vi "iLogDemostrator.vi"() -> ()   [LabVIEW 2019]
uses:
  ByteQXAPIBase/TypeDef/Test.ctl
  ByteQXAPIBase/TypeDef/Asset.ctl
  ByteQXAPIBase/TypeDef/Step.ctl
  ByteQXAPIBase/ByteQXAPIBase.lvclass
  ByteQXAPIBase/iLOGAcquisition/Acquisitions.ctl
  <vilib>/numeric/Random Number (Range) U64.vi
  <vilib>/numeric/sub_Random U32.vi
  <vilib>/Bytelabs/ByteSimpleQ/ByteSimpleQ/ByteSimpleQ.lvlib
panel:
  out "Single Asset":string
  in  "Begin Acq":bool
  in  "Channels":cluster{"Channel Name":string, "Delete":bool}[](array[cluster])
  in  "LogSingle":bool
  in  "Asset Code":string="BNC0001"
  in  "Start":bool
  out "Values":cluster{"Channel Name":string, "Value":dbl}[](array[cluster])
  out "Waveform Chart":T1(graph)
  in  "Stop":bool
  out "Title":string
  in  "Channels":cluster{"Channel Name":string, "Delete":bool}[](array[cluster])
  in  "Select Asset":i32(ring) items=["BNC0001"]
  out "InfoStep":string caption="Step Information"
  in  "Select Step":i32(ring) items=["Warm-up"=183, "Full loaded test cycle"=184]
  out "InfoTest":string caption="Test Information"
  in  "Inizia Test":bool
  in  "Select Test":i32(ring) items=["T0008 - Richiesta prova test di durata"=69, "T0003 - Endurance test 19/02/2025"=64, "T0021 - Prova da form"=82, "T0018 - Prova da form"=79, "T0001 - Endurance test 19/02/2025"=62, "T0019 - Prova da form"=80, "T0022 - Test Fan Plan"=83, "T0002 - Endurance test 19/02/2025"=63]
  in  "GetTests":bool
  in  "Starting Date":timestamp format="%<%x>T"
  in  "Workstation":u16(ring) items=["Sala gialla", "POST 1"]
  in  "Exit":bool
  in  "Home":bool
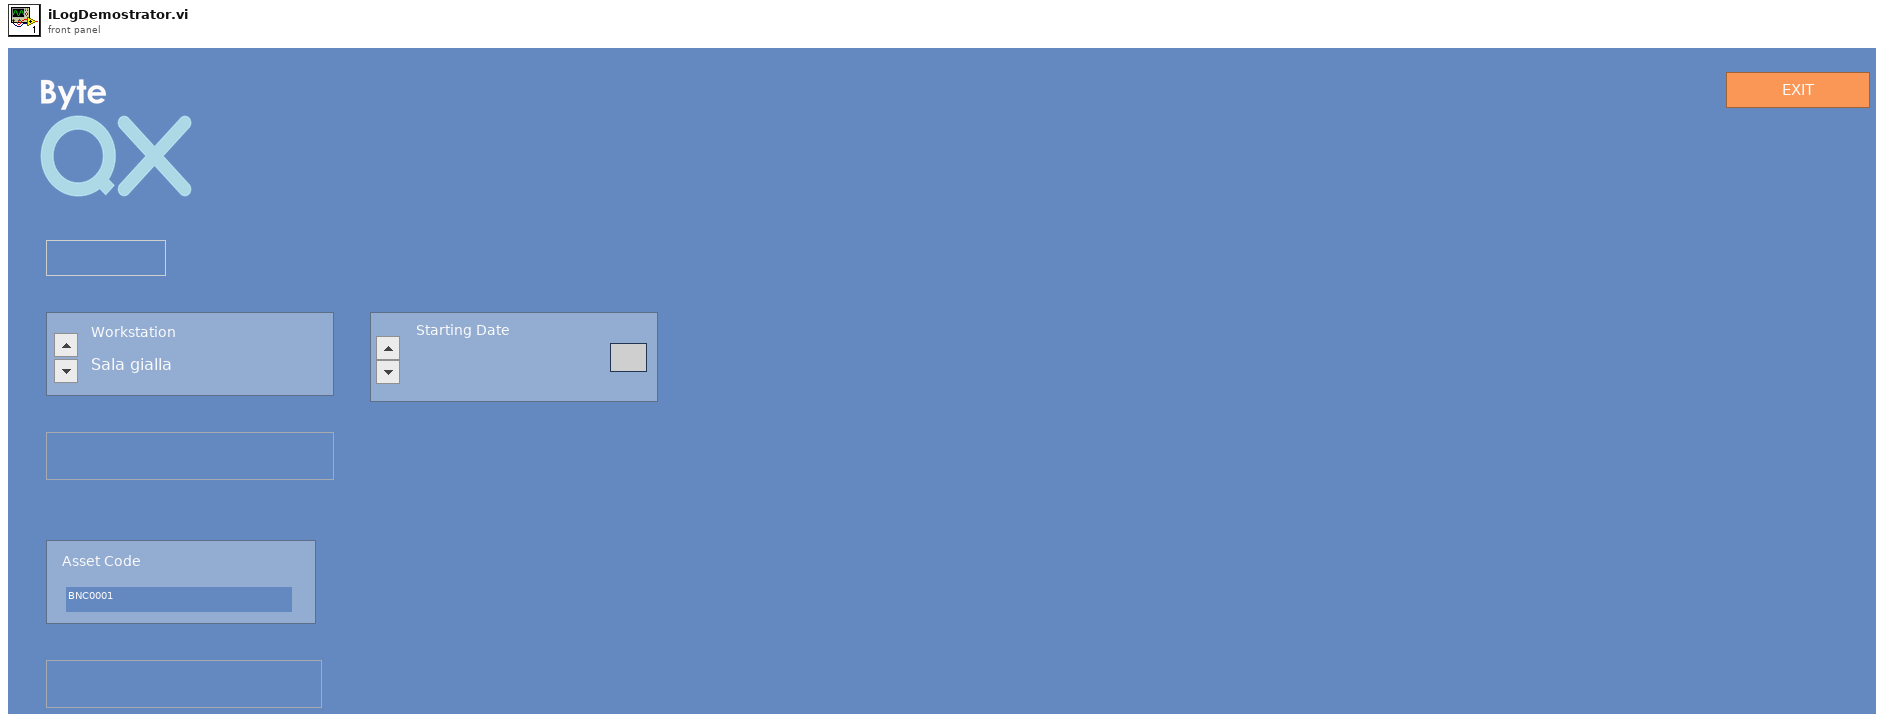
[diagram p1: front panel]
types:
  T1 = cluster{"Graph[0]":u64, "Graph[1]":u64, "Graph[2]":u64, "Graph[3]":u64, "Graph[4]":u64, "Graph[5]":u64, "Graph[6]":u64, "Graph[7]":u64, "Graph[8]":u64, "Graph[9]":u64, "Graph[10]":u64, "Graph[11]":u64, "Graph[12]":u64, "Graph[13]":u64, "Graph[14]":u64, "Graph[15]":u64, "Graph[16]":u64, "Graph[17]":u64, "Graph[18]":u64, "Graph[19]":u64, "Graph[20]":u64, "Graph[21]":u64, "Graph[22]":u64, "Graph[23]":u64, "Graph[24]":u64, "Graph[25]":u64, "Graph[26]":u64, "Graph[27]":u64, "Graph[28]":u64, "Graph[29]":u64, "Graph[30]":u64, "Graph[31]":u64, "Graph[32]":u64, "Graph[33]":u64, "Graph[34]":u64, "Graph[35]":u64, "Graph[36]":u64, "Graph[37]":u64, "Graph[38]":u64, "Graph[39]":u64, "Graph[40]":u64, "Graph[41]":u64, "Graph[42]":u64, "Graph[43]":u64, "Graph[44]":u64, "Graph[45]":u64, "Graph[46]":u64, "Graph[47]":u64, "Graph[48]":u64, "Graph[49]":u64}
  T2 = cluster{"Begin Acq":refnum<vi>, "Channels":refnum<vi>, "Single Asset":refnum<vi>}
  T3 = cluster{"Title":refnum<vi>, "Stop":refnum<vi>, "Values":refnum<vi>, "Start":refnum<vi>, "Waveform Chart":refnum<vi>}
  T4 = typedef "ByteQXWebAPI.lvlib/ByteQXAPIBase.lvclass/Step.ctl" = cluster{"id":i32, "descrizione":string, "prova":cluster{"slug":string}, "assets":T5[], "criterio_accettazione":string, "valore_criterio_accettazione_max":dbl, "valore_criterio_accettazione_min":dbl, "udm_criterio_accettazione":string, "duration_prova":string, "udm_duration_prova":string, "valore_prova":dbl, "ordine":i32, "user":i32, "link_automation":string, "instruction_automation":string, "data_completamento_checklist":timestamp, "outcome":bool, "step_type":string, "channels":string[]}
  T5 = typedef "ByteQXWebAPI.lvlib/ByteQXAPIBase.lvclass/Asset.ctl" = cluster{"descrizione":string, "slug":string, "id":i32}
  T6 = cluster{"Select Test":refnum<vi>, "InfoTest":refnum<vi>, "Inizia Test":refnum<vi>, "Select Step":refnum<vi>, "InfoStep":refnum<vi>, "Select Asset":refnum<vi>, "Channels":refnum<vi>}
  T7 = typedef "ByteQXWebAPI.lvlib/ByteQXAPIBase.lvclass/Test.ctl" = cluster{"titolo":string, "descrizione":string, "statoprova":string, "assets":T5[], "id":i32, "data_apertura_prova":timestamp, "slug":string}
  T8 = cluster{"Workstation":refnum<vi>, "Starting Date":refnum<vi>, "GetTests":refnum<vi>, "Asset Code":refnum<vi>, "LogSingle":refnum<vi>}
  T9 = cluster{"ByteQXAPIBase in":refnum<class "ByteQXAPIBase.lvclass">, "Array dei Test":T7[], "InfoTest":string, "InfoStep":string, "Steps Array":T4[], "queue out":refnum<queue>, "Title":string}
  T10 = cluster{"Single":cluster{"Begin Acq":refnum<vi>, "Channels":refnum<vi>, "Single Asset":refnum<vi>}, "Home":cluster{"Workstation":refnum<vi>, "Starting Date":refnum<vi>, "GetTests":refnum<vi>, "Asset Code":refnum<vi>, "LogSingle":refnum<vi>}, "Test":cluster{"Select Test":refnum<vi>, "InfoTest":refnum<vi>, "Inizia Test":refnum<vi>, "Select Step":refnum<vi>, "InfoStep":refnum<vi>, "Select Asset":refnum<vi>, "Channels":refnum<vi>}, "Running":cluster{"Title":refnum<vi>, "Stop":refnum<vi>, "Values":refnum<vi>, "Start":refnum<vi>, "Waveform Chart":refnum<vi>}}
  T11 = cluster{"Values":cluster{"Channel Name":string, "Value":dbl}[], "ByteQXAPIBase in":refnum<class "ByteQXAPIBase.lvclass">, "slug":string, "Step Id":i32, "AssetCode":string, "Graph":u64[], "Waveform Chart":refnum<vi>}
  T12 = cluster{"Graph[0]":u64, "Graph[1]":u64, "Graph[2]":u64, "Graph[3]":u64, "Graph[4]":u64, "Graph[5]":u64, "Graph[6]":u64, "Graph[7]":u64, "Graph[8]":u64, "Graph[9]":u64, "Graph[10]":u64, "Graph[11]":u64, "Graph[12]":u64, "Graph[13]":u64, "Graph[14]":u64, "Graph[15]":u64, "Graph[16]":u64, "Graph[17]":u64, "Graph[18]":u64, "Graph[19]":u64, "Graph[20]":u64, "Graph[21]":u64, "Graph[22]":u64, "Graph[23]":u64, "Graph[24]":u64, "Graph[25]":u64, "Graph[26]":u64, "Graph[27]":u64, "Graph[28]":u64, "Graph[29]":u64, "Graph[30]":u64, "Graph[31]":u64, "Graph[32]":u64, "Graph[33]":u64, "Graph[34]":u64, "Graph[35]":u64, "Graph[36]":u64, "Graph[37]":u64, "Graph[38]":u64, "Graph[39]":u64, "Graph[40]":u64, "Graph[41]":u64, "Graph[42]":u64, "Graph[43]":u64, "Graph[44]":u64, "Graph[45]":u64, "Graph[46]":u64, "Graph[47]":u64, "Graph[48]":u64, "Graph[49]":u64}[]
  T13 = cluster{"ByteQXAPIBase in":refnum<class "ByteQXAPIBase.lvclass">, "slug":string, "Channels":string[], "Step Id":i32, "AssetCode":string}
  T14 = cluster{"Workstation":u16, "Starting Date":timestamp, "Select Test":i32, "Select Step":i32, "Select Asset":i32, "Channels":cluster{"Channel Name":string, "Delete":bool}[], "Asset Code":string, "Channels":cluster{"Channel Name":string, "Delete":bool}[]}
  T15 = typedef "ByteQXWebAPI.lvlib/ByteQXAPIBase.lvclass/Acquisitions.ctl" = cluster{"timestamp":timestamp, "channels":cluster{"name":string, "value":dbl}[]}
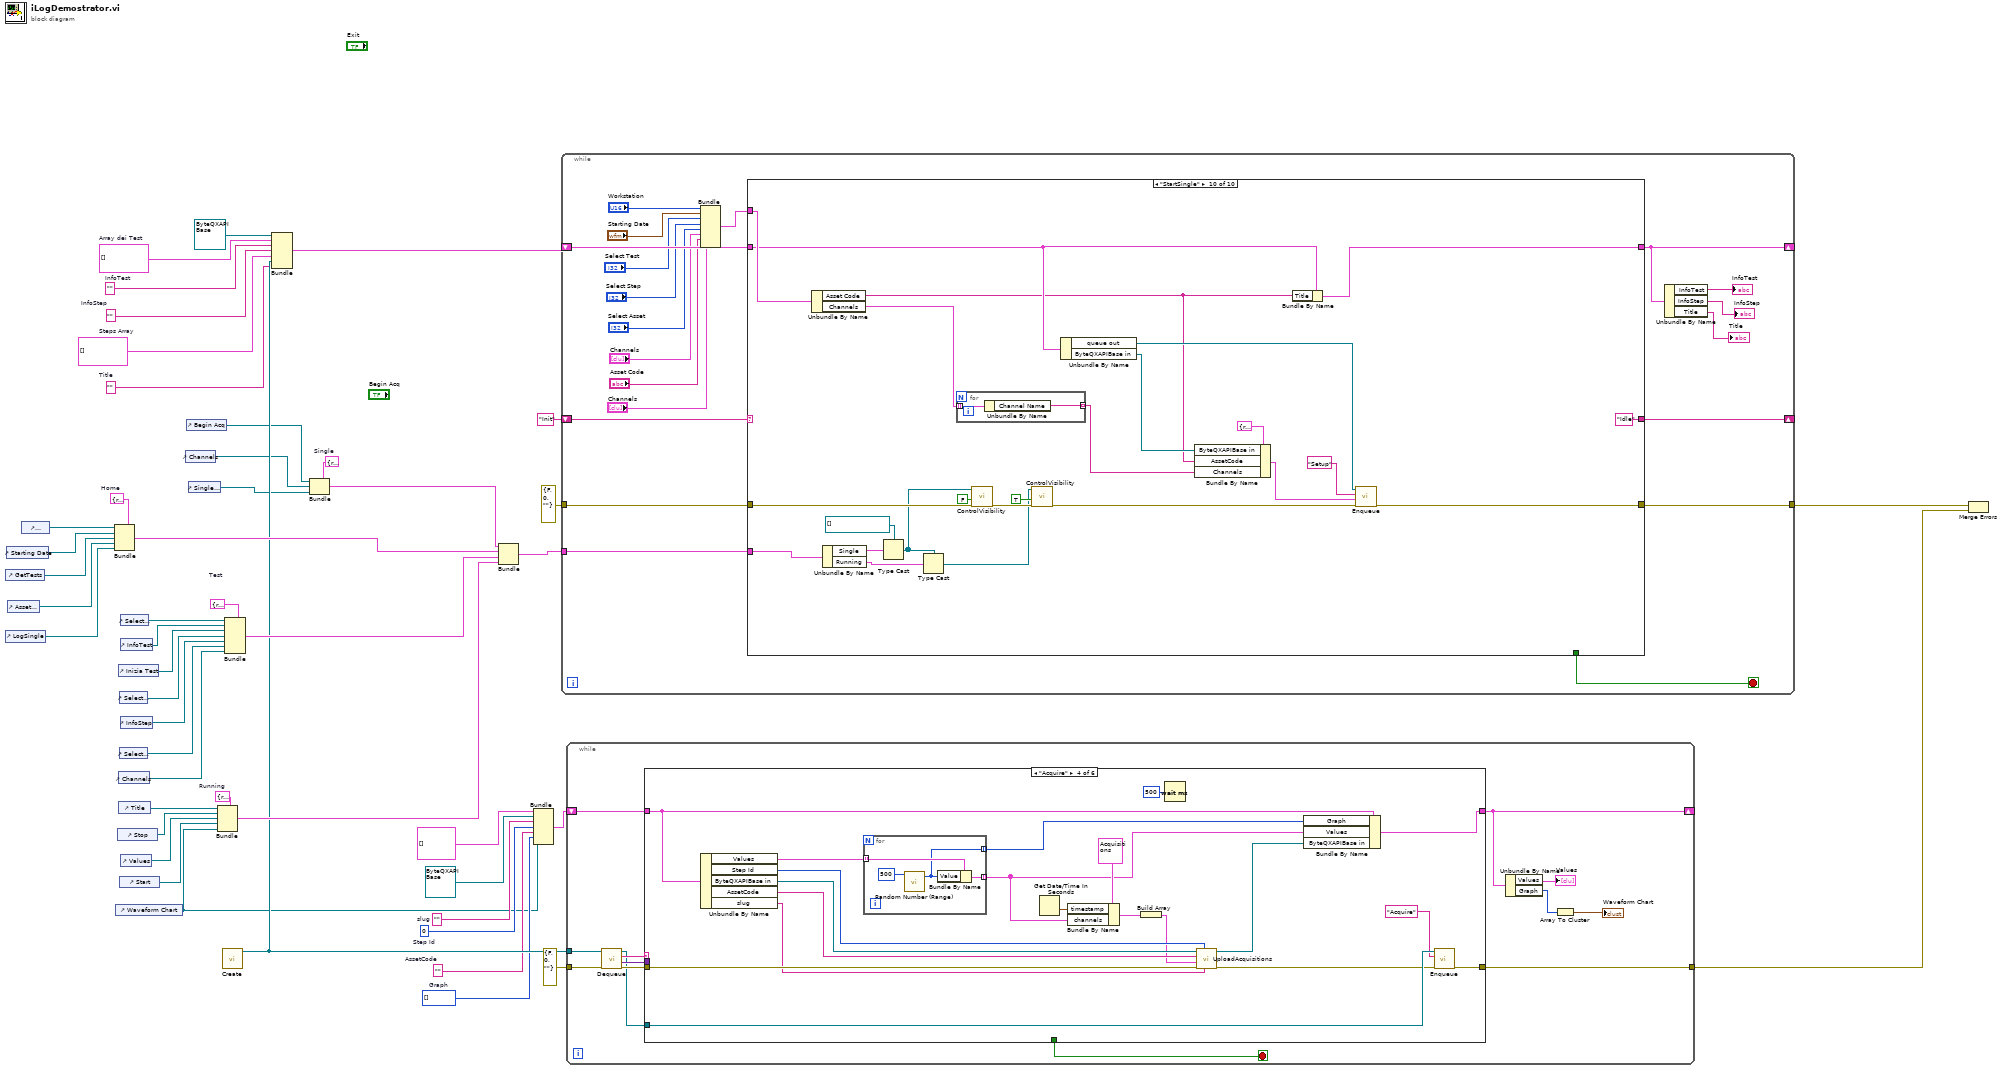
[diagram p0: block diagram]
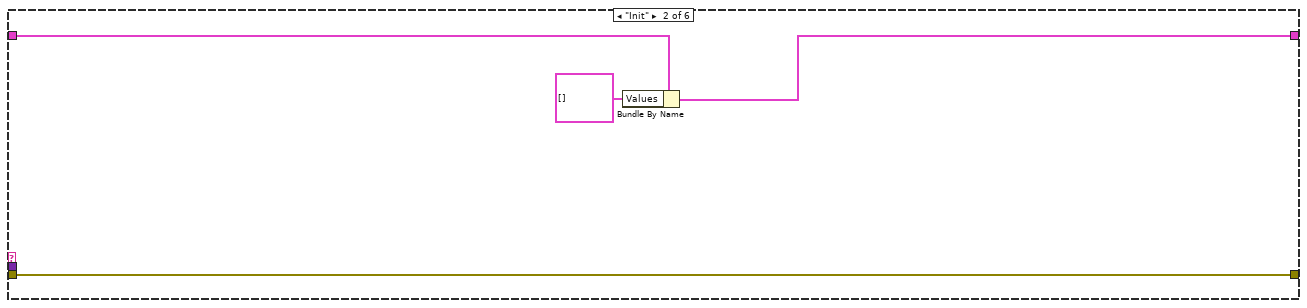
[diagram p3: hidden frame]
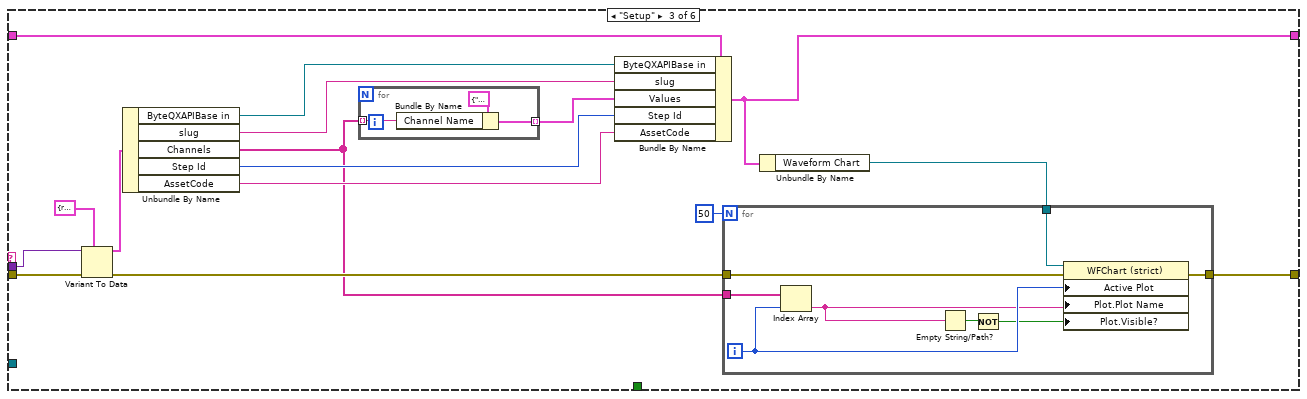
[diagram p4: hidden frame]
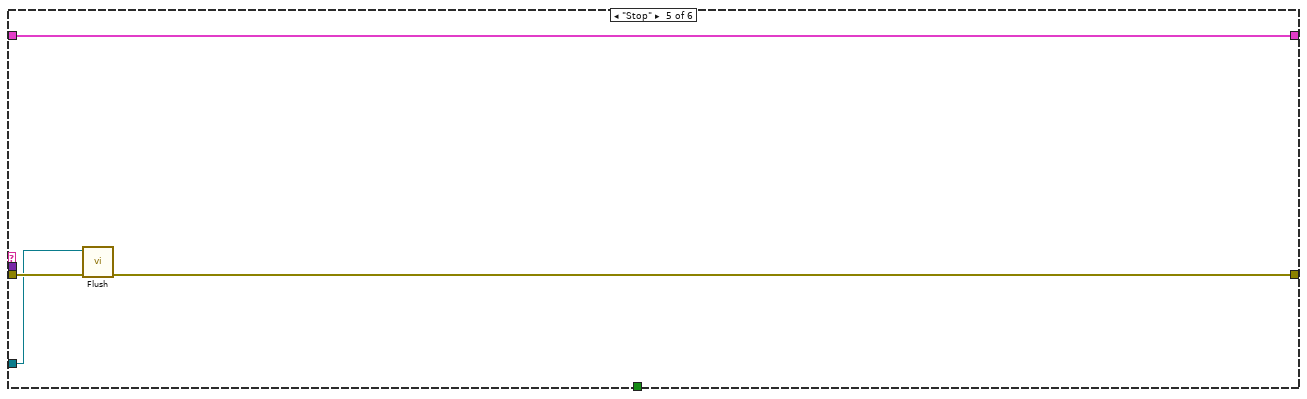
[diagram p5: hidden frame]
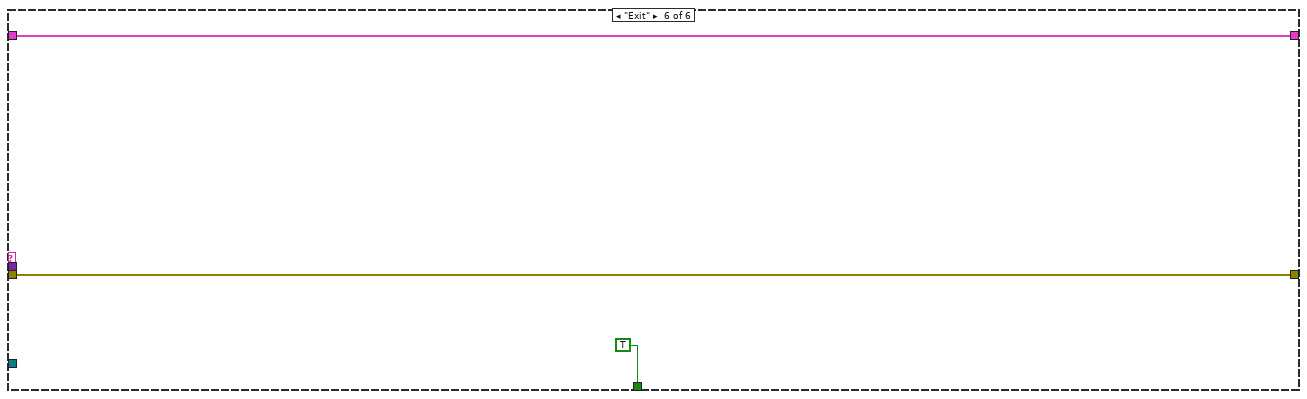
[diagram p6: hidden frame]
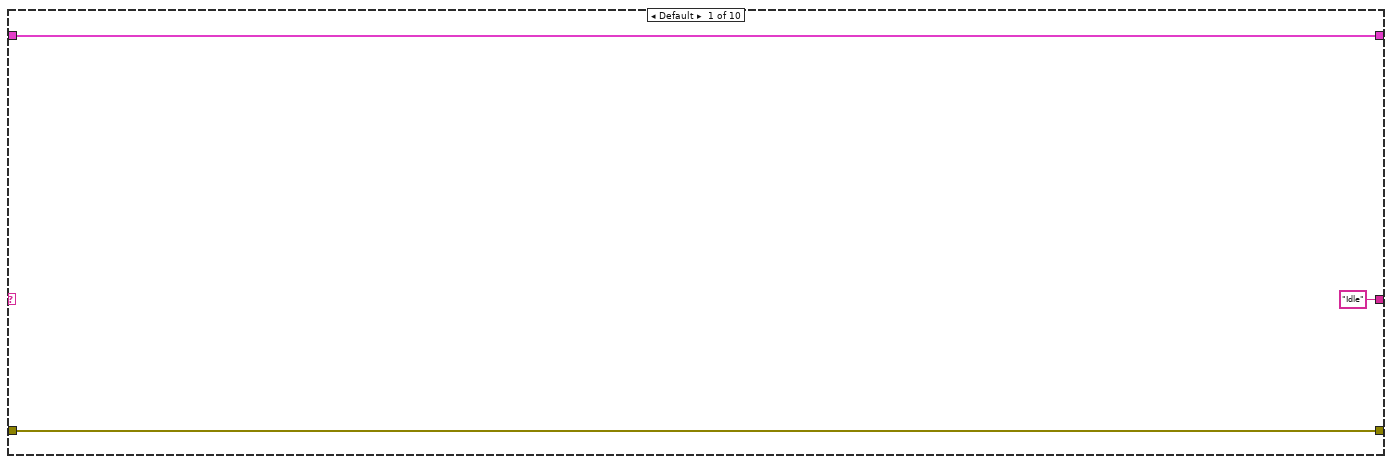
[diagram p7: hidden frame]
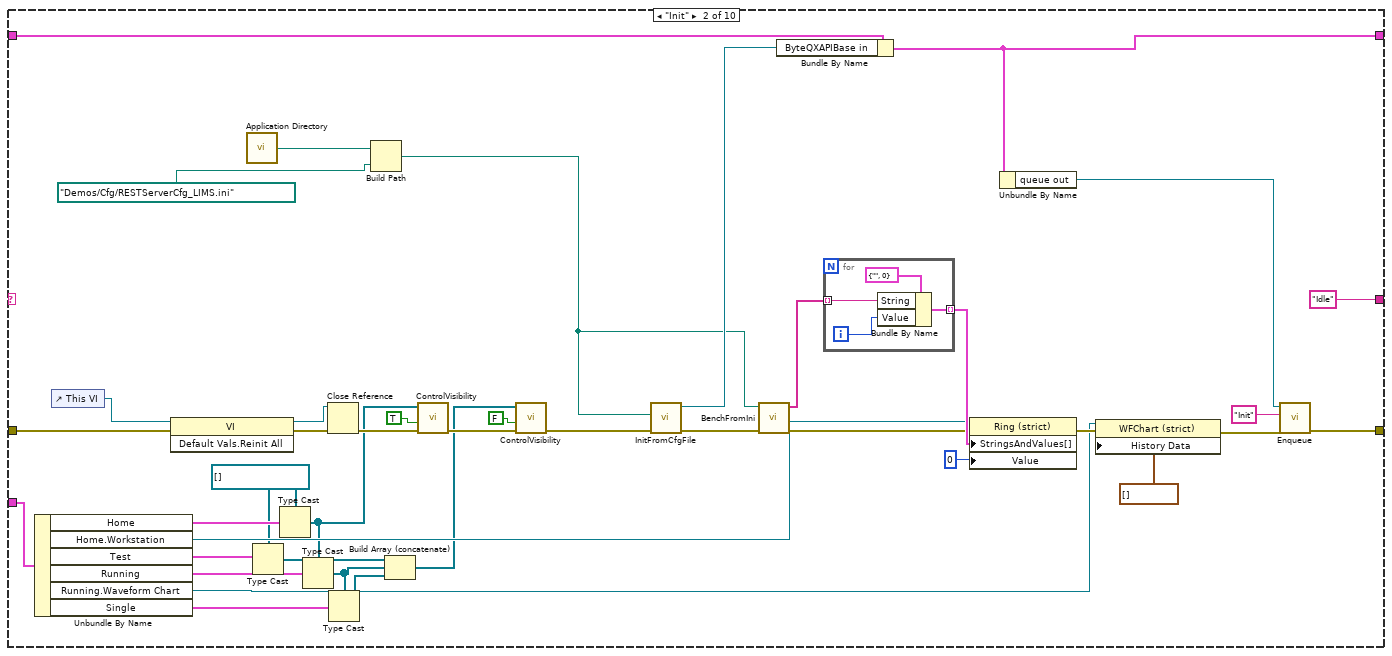
[diagram p8: hidden frame]
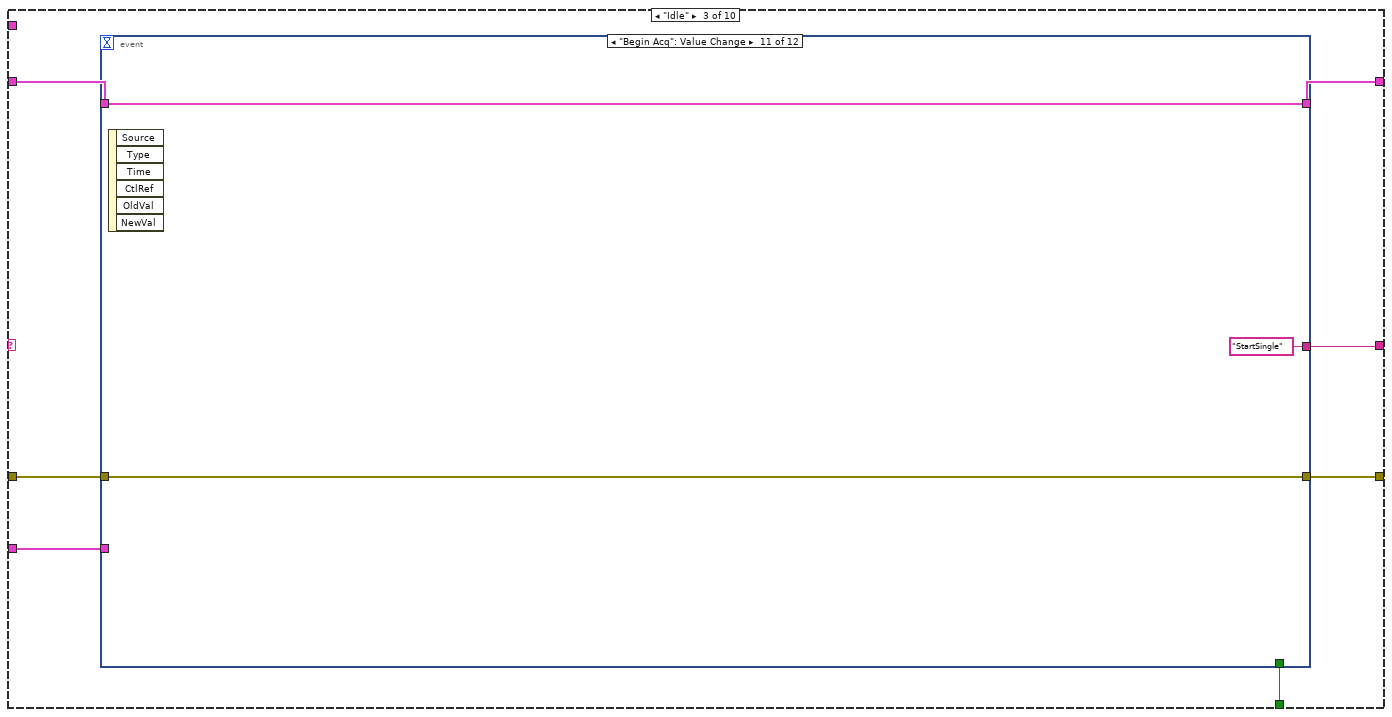
[diagram p9: hidden frame]
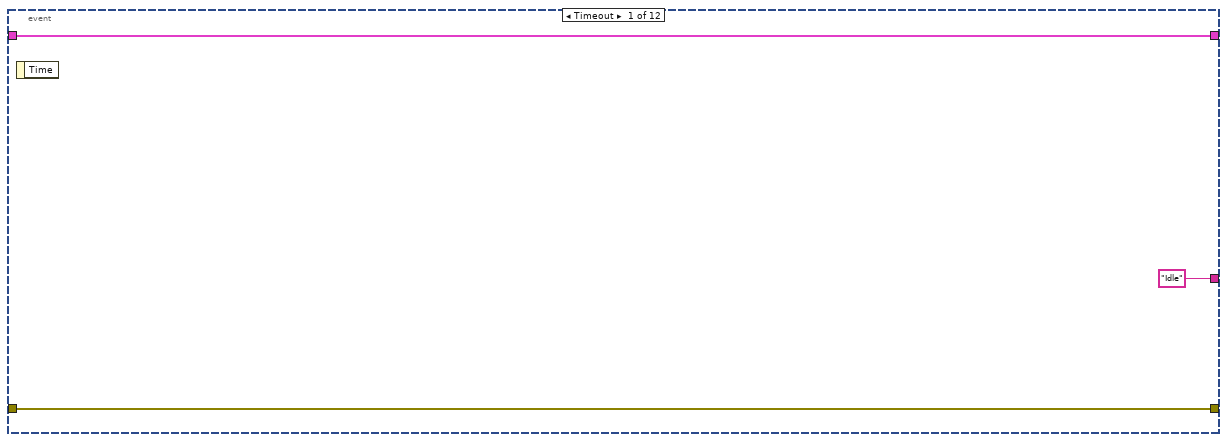
[diagram p10: hidden frame]
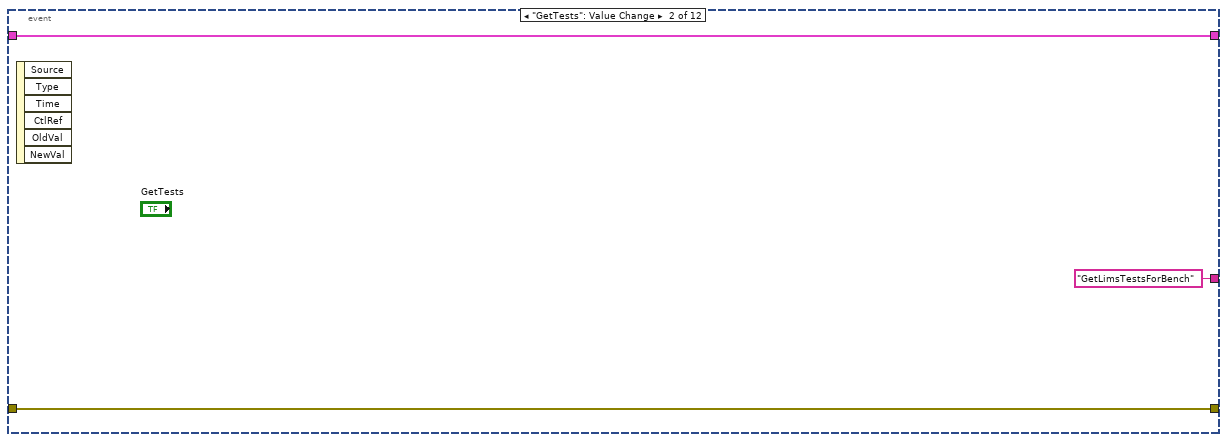
[diagram p11: hidden frame]
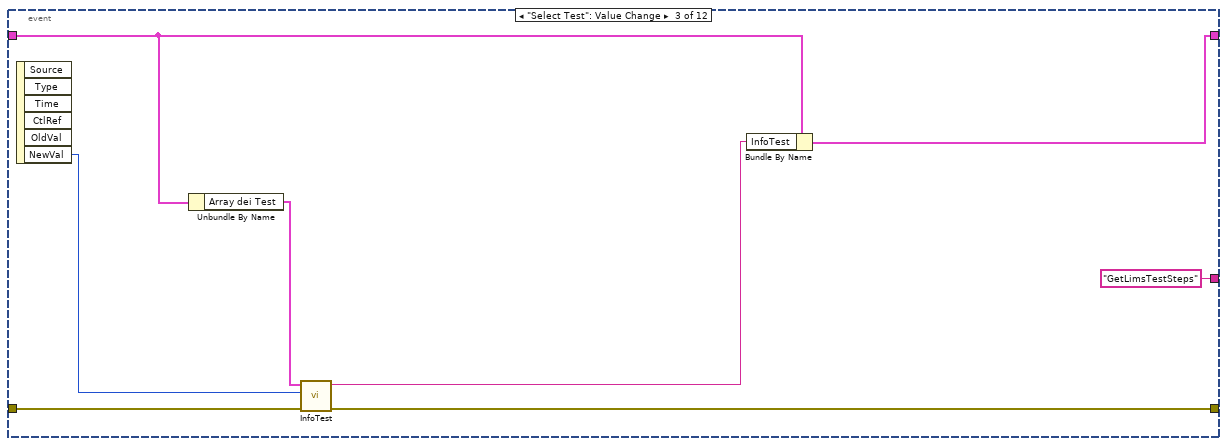
[diagram p12: hidden frame]
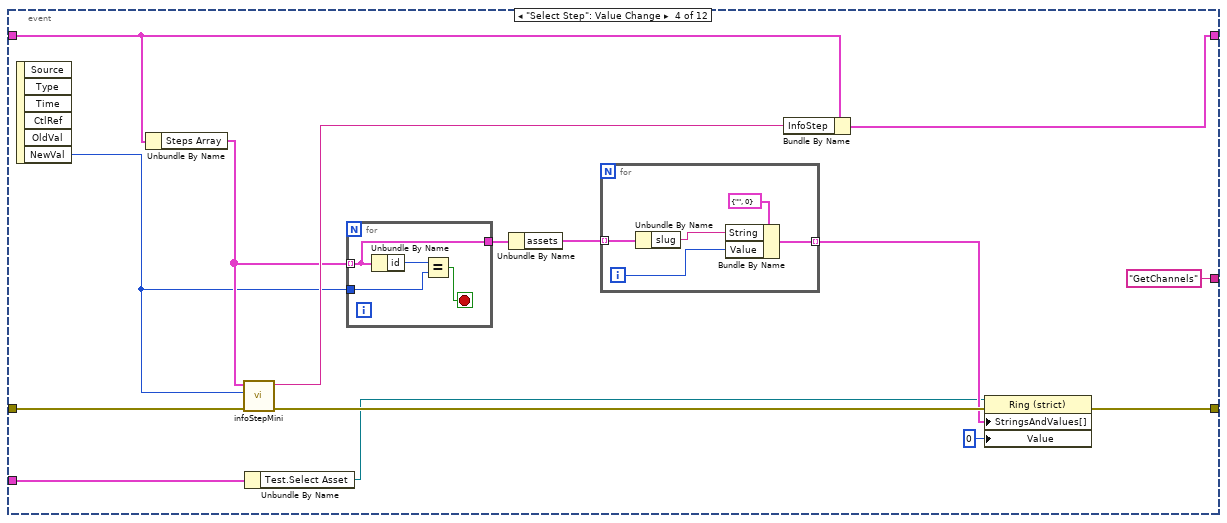
[diagram p13: hidden frame]
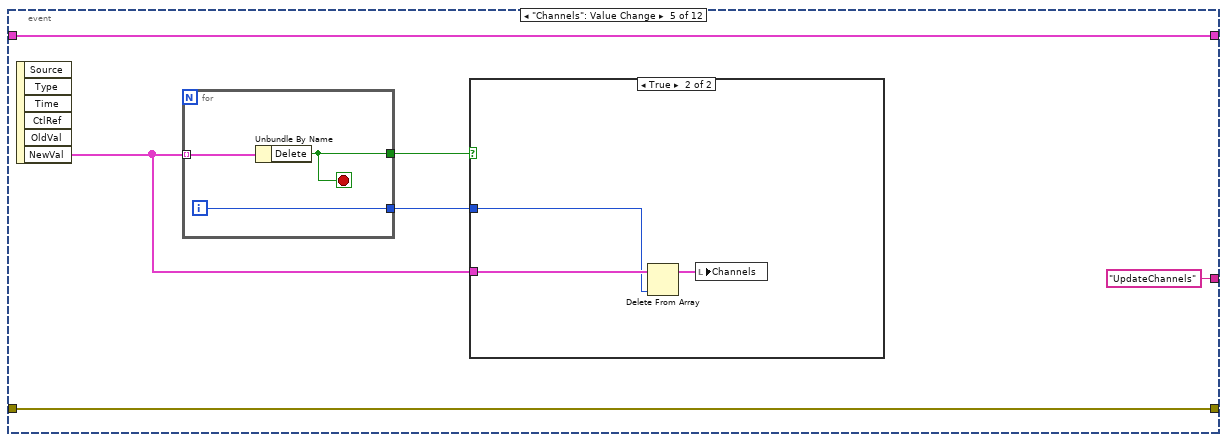
[diagram p14: hidden frame]
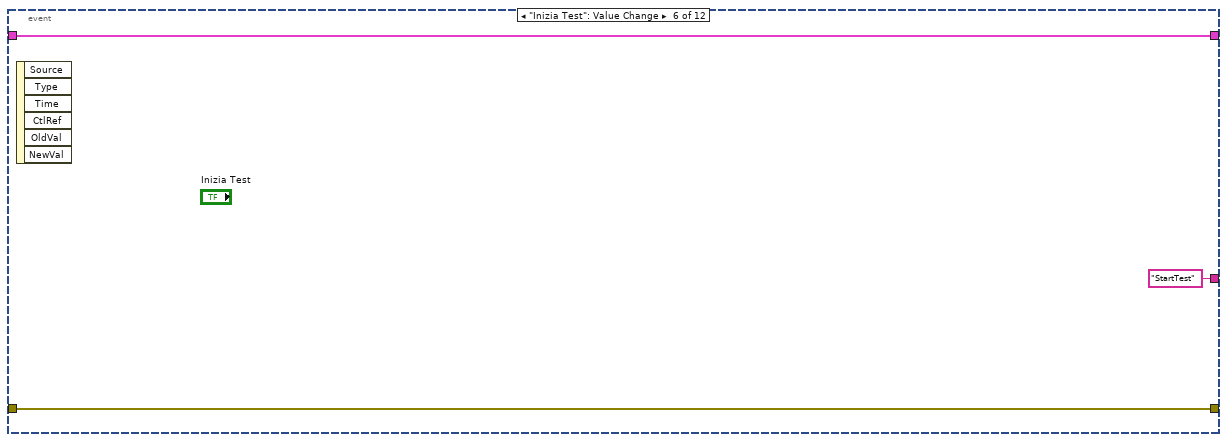
[diagram p16: hidden frame]
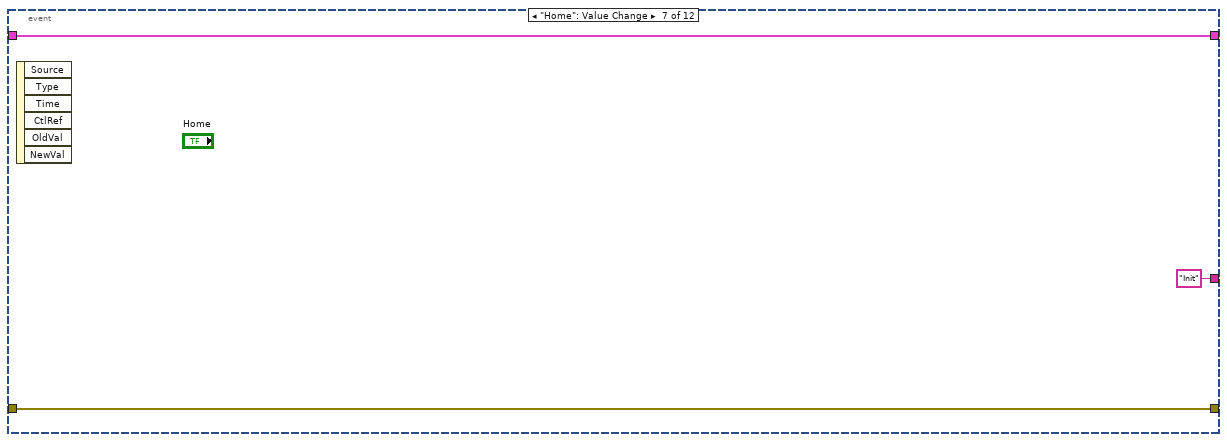
[diagram p17: hidden frame]
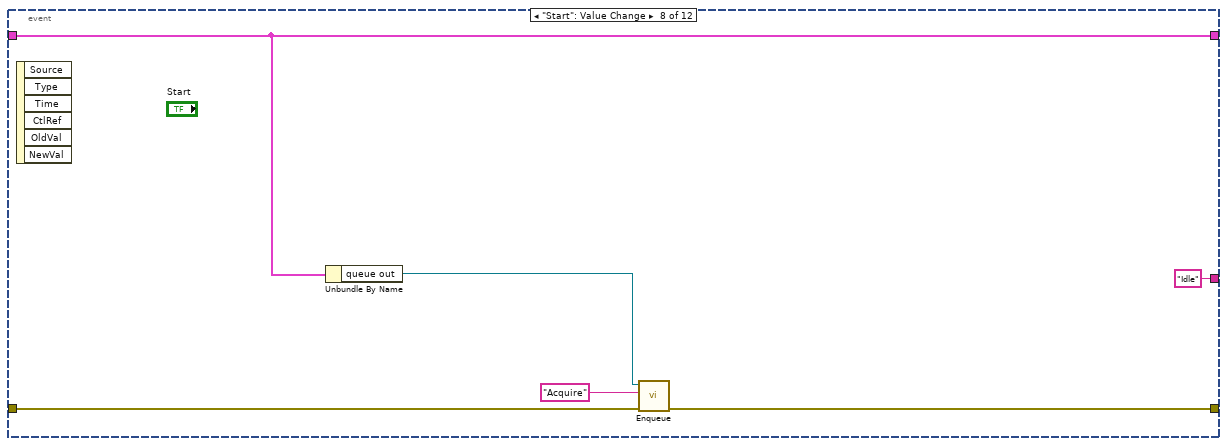
[diagram p18: hidden frame]
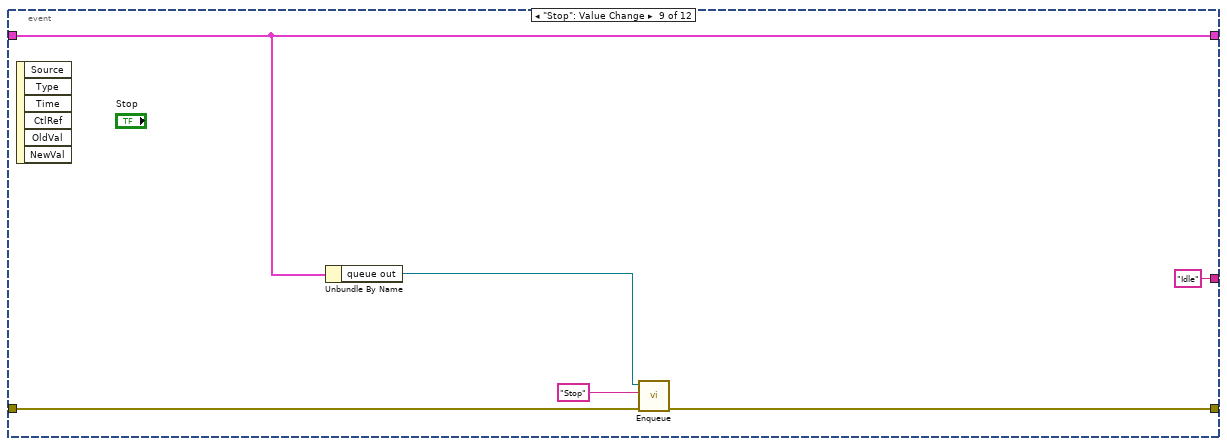
[diagram p19: hidden frame]
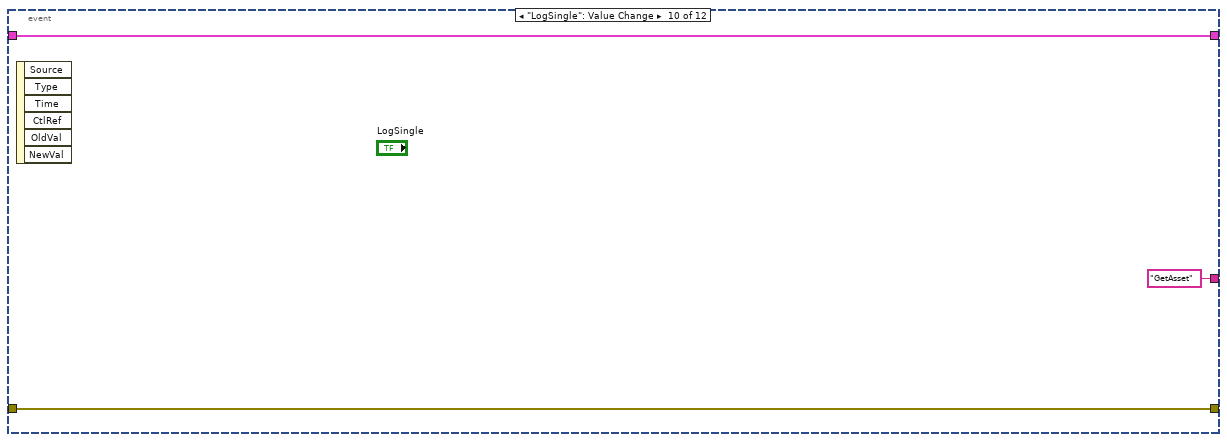
[diagram p20: hidden frame]
diagram:
  w1 = ""  # Title
  w6 = T2 {"Begin Acq"=refnum, "Channels"=refnum, "Single Asset"=refnum}  # Single
  w14 = u64[] []  # Graph
  w15 = ""  # AssetCode
  w16 = 0  # Step Id
  w17 = ""  # slug
  w24 = T3 {"Title"=refnum, "Stop"=refnum, "Values"=refnum, "Start"=refnum, "Waveform Chart"=refnum}  # Running
  w29 = T4[] []  # Steps Array
  w30 = T6 {"Select Test"=refnum, "InfoTest"=refnum, "Inizia Test"=refnum, "Select Step"=refnum, "InfoStep"=refnum, "Select Asset"=refnum, "Channels"=refnum}  # Test
  w33 = ""  # InfoStep
  w34 = ""  # InfoTest
  w35 = T7[] []  # Array dei Test
  w36 = T8 {"Workstation"=refnum, "Starting Date"=refnum, "GetTests"=refnum, "Asset Code"=refnum, "LogSingle"=refnum}  # Home
  n1 = control-ref of="GetTests"() -> (w39:refnum<vi>)
  n2 = control-ref of="LogSingle"() -> (w3:refnum<vi>)
  n3 = control-ref of="Starting Date"() -> (w37:refnum<vi>)
  n4 = control-ref of="Asset Code"() -> (w4:refnum<vi>)
  n5 = control-ref of="Workstation"() -> (w45:refnum<vi>)
  n6 = Bundle(cluster=w36, "Workstation"=w45, "Starting Date"=w37, "GetTests"=w39, "Asset Code"=w4, "LogSingle"=w3) -> (w44:T8)
  n7 = control-ref of="Waveform Chart"() -> (w11:refnum<vi>)
  n8 = control-ref of="Stop"() -> (w23:refnum<vi>)
  n9 = control-ref of="Inizia Test"() -> (w38:refnum<vi>)
  n10 = control-ref of="Channels"() -> (w27:refnum<vi>)
  n11 = control-ref of="Title"() -> (w26:refnum<vi>)
  n12 = control-ref of="Select Step"() -> (w32:refnum<vi>)
  n13 = control-ref of="Select Asset"() -> (w28:refnum<vi>)
  n14 = control-ref of="Start"() -> (w12:refnum<vi>)
  n15 = control-ref of="Select Test"() -> (w42:refnum<vi>)
  n16 = control-ref of="InfoTest"() -> (w41:refnum<vi>)
  n17 = control-ref of="InfoStep"() -> (w31:refnum<vi>)
  n18 = control-ref of="Values"() -> (w13:refnum<vi>)
  n19 = control-ref of="Channels"() -> (w7:refnum<vi>)
  n20 = control-ref of="Begin Acq"() -> (w8:refnum<vi>)
  n21 = control-ref of="Single Asset"() -> (w2:refnum<vi>)
  n22 = Bundle(cluster=w24, "Title"=w26, "Stop"=w23, "Values"=w13, "Start"=w12, "Waveform Chart"=w11) -> (w25:T3)
  n23 = call <vilib>:"Create.vi"() -> ("queue out"=w21:refnum<queue>)  [unwired: 9 in, 2 out]
  n24 = Bundle(cluster=w30, "Select Test"=w42, "InfoTest"=w41, "Inizia Test"=w38, "Select Step"=w32, "InfoStep"=w31, "Select Asset"=w28, "Channels"=w27) -> (w40:T6)
  n25 = Bundle("ByteQXAPIBase in"=refnum<class "ByteQXAPIBase.lvclass"> refnum, "Array dei Test"=w35, "InfoTest"=w34, "InfoStep"=w33, "Steps Array"=w29, "queue out"=w21, "Title"=w1) -> (w48:T9)  [unwired: 1 in]
  n26 = Bundle(cluster=w6, "Begin Acq"=w8, "Channels"=w7, "Single Asset"=w2) -> (w5:T2)
  n27 = Bundle("Single"=w5, "Home"=w44, "Test"=w40, "Running"=w25) -> (w43:T10)  [unwired: 1 in]
  n28 = Bundle("Values"=cluster{"Channel Name":string, "Value":dbl}[] [], "ByteQXAPIBase in"=refnum<class "ByteQXAPIBase.lvclass"> refnum, "slug"=w17, "Step Id"=w16, "AssetCode"=w15, "Graph"=w14, "Waveform Chart"=w11) -> (w22:T11)  [unwired: 1 in]
  n29 = while {
    shift-right: [w59] -> _
    shift-left: w48 -> [w69]
    shift-right: [w64] -> _
    shift-left: "Init" -> [w68]
    tunnel: errorcluster {"status"=FALSE, "code"=0, "source"=""} ("error in (no error)") -> [w67]
    tunnel: w43 -> [w66]
    tunnel: [w65] -> w10
    stop <- w55 stop-if-true
    n30 = Bundle("Workstation"="Workstation", "Starting Date"="Starting Date", "Select Test"="Select Test", "Select Step"="Select Step", "Select Asset"="Select Asset", "Channels"="Channels", "Asset Code"="Asset Code", "Channels"="Channels") -> (w61:T14)  [unwired: 1 in]
    n31 = case shown="\"StartSingle\"" w68 {
      tunnel: w69 -> [w71 w106 w121 w219 w264 w285 w301 w316 w383 w399]
      tunnel: w67 -> [w72 w108 w122 w221 w262 w292 w307 w348 w378 w411]
      tunnel: [w71 w83 w120 w217 w263 w284 w300 w315 w382 w403] -> w59
      tunnel: w66 -> [_ w91 w123 w234 w257 w291 w306 w351 w376 w410]
      tunnel: [w72 w81 w119 w213 w254 w282 w298 w325 w385 w397] -> w65
      tunnel: ["Idle" "Idle" w118 "GetLimsTestSteps" "GetChannels" "Idle" "Idle" "Idle" "Idle" "Idle"] -> w64
      tunnel: w61 -> [_ _ _ w222 w265 w289 w311 w349 w387 w404]
      tunnel: [_ _ w117 _ _ _ _ _ _ _] -> w55
      frame Default {
      }
      frame "Init" {
        w88 = refnum<vi>[] [] ("Controls")
        n32 = Unbundle By Name(w91) -> ("Home"=w92:T8, "Home.Workstation"=w90:refnum<vi>, "Test"=w89:T6, "Running"=w87:T3, "Running.Waveform Chart"=w78:refnum<vi>, "Single"=w75:T2)
        n33 = control-ref of="This VI"() -> (w107:refnum<vi>)
        n34 = invoke class="VI" method="Default Vals.Reinit All"(reference=w107, error in=w108) -> (reference out=w110:refnum<vi>, error out=w109:errorcluster)  [unwired: 1 in, 1 out]
        n35 = call <vilib>:"Application Directory.vi"() -> ("Application Directory"=w112:path)
        n36 = Type Cast(type=w88, x=w89) -> (*(type *) &x=w85:refnum<vi>[])
        n37 = Type Cast(type=w88, x=w92) -> (*(type *) &x=w86:refnum<vi>[])
        n38 = Type Cast(type=w86, x=w87) -> (*(type *) &x=w74:refnum<vi>[])
        n39 = Close Reference(reference=w110, error in (no error)=w109) -> (error out=w98:errorcluster)
        n40 = Type Cast(type=w74, x=w75) -> (*(type *) &x=w73:refnum<vi>[])
        n41 = Build Path(base path=w112, name or relative path=path "Demos/Cfg/RESTServerCfg_LIMS.ini") -> (appended path=w103:path)
        n42 = Build Array (concatenate)(w85, w74, w73) -> (w84:refnum<vi>[])
        n43 = call "ControlVisibility.vi"("error in (no error)"=w98, "Visible"=TRUE, "Controls"=w86) -> ("error out"=w96:errorcluster)  [unwired: 8 in]
        n44 = call "ControlVisibility.vi"("error in (no error)"=w96, "Visible"=FALSE, "Controls"=w84) -> ("error out"=w94:errorcluster)  [unwired: 8 in]
        n45 = call "InitFromCfgFile.vi"("error in (no error)"=w94, "configuration file path"=w103) -> ("error out"=w104:errorcluster, "ByteQXAPIBase out"=w105:refnum<class "ByteQXAPIBase.lvclass">)  [unwired: 8 in]
        n46 = call "BenchFromIni.vi"("error in (no error)"=w104, "configuration file path"=w103) -> ("error out"=w99:errorcluster, "Array"=w102:string[])  [unwired: 8 in]
        n47 = Bundle By Name(cluster=w106, "ByteQXAPIBase in"=w105) -> (w83:T9)
        n48 = for {
          tunnel: w102 -> [w115] mode=indexing
          tunnel: [w113] -> w100 mode=indexing
          i -> [w114]
          n49 = Bundle By Name(cluster=cluster{"String":string, "Value":u16} {"String"="", "Value"=0} ("Cluster"), "String"=w115, "Value"=w114) -> (w113:cluster{"String":string, "Value":u16})
        }
        n50 = property class="Ring (strict)"(reference=w90, error in=w99, "StringsAndValues[]"=w100, "Value"=u16 0) -> (error out=w79:errorcluster)  [unwired: 1 out]
        n51 = Unbundle By Name(w83) -> ("queue out"=w82:refnum<queue>)
        n52 = property class="WFChart (strict)"(reference=w78, error in=w79, "History Data"=T12 []) -> (error out=w77:errorcluster)  [unwired: 1 out]
        n53 = call <vilib>:"Enqueue.vi"("error in (no error)"=w77, "message"="Init", "queue in"=w82) -> ("error out"=w81:errorcluster)  [unwired: 6 in, 2 out]
      }
      frame "Idle" {
        n54 = event shown="[10] \"Begin Acq\": Value Change" {
          selector: _ -> [_ _ _ _ _ _ _ _ _ _ _ _]
          dyn-events: _ -> [_ _ _ _ _ _ _ _ _ _ _ _]
          timeout: _ -> [_ _ _ _ _ _ _ _ _ _ _ _]
          tunnel: w123 -> [_ _ _ w143 _ _ _ _ _ _ _ _]
          tunnel: w122 -> [w125 w128 w137 w152 w166 w175 w178 w185 w191 w193 w196 w202]
          tunnel: w121 -> [w126 w129 w134 w151 w167 w176 w179 w183 w189 w194 w197 w200]
          tunnel: [w126 w129 w133 w150 w167 w176 w179 w183 w189 w194 w197 w200] -> w120
          tunnel: [w125 w128 w131 w140 w166 w175 w178 w184 w190 w193 w196 w201] -> w119
          tunnel: ["Idle" "GetLimsTestsForBench" "GetLimsTestSteps" "GetChannels" "UpdateChannels" "StartTest" "Init" "Idle" "Idle" "GetAsset" "StartSingle" _] -> w118
          tunnel: [_ _ _ _ _ _ _ _ _ _ _ TRUE] -> w117
          event Timeout {
            n55 = event-data() -> ()  [unwired: 1 in, 1 out]
          }
          event "GetTests": Value Change {
            n56 = event-data() -> ()  [unwired: 1 in, 6 out]
          }
          event "Select Test": Value Change {
            n57 = event-data() -> ("NewVal"=w135:i32)  [unwired: 1 in, 5 out]
            n58 = Unbundle By Name(w134) -> ("Array dei Test"=w136:T7[])
            n59 = call "InfoTest.vi"("error in"=w137, "Seleziona Test"=w135, "TestForBenchArray"=w136) -> ("error out"=w131:errorcluster, "Info Test"=w132:string)  [unwired: 7 in]
            n60 = Bundle By Name(cluster=w134, "InfoTest"=w132) -> (w133:T9)
          }
          event "Select Step": Value Change {
            n61 = event-data() -> ("NewVal"=w146:i32)  [unwired: 1 in, 5 out]
            n62 = Unbundle By Name(w151) -> ("Steps Array"=w147:T4[])
            n63 = call "infoStepMini.vi"("error in (no error)"=w152, "StepId"=w146, "Array"=w147) -> ("error out"=w141:errorcluster, "Info Test"=w149:string)  [unwired: 7 in]
            n64 = Unbundle By Name(w143) -> ("Test.Select Asset"=w138:refnum<vi>)
            n65 = for {
              tunnel: w147 -> [w158] mode=indexing
              tunnel: w146 -> [w160]
              tunnel: [w158] -> w145
              stop <- w159 stop-if-true
              n66 = Unbundle By Name(w158) -> ("id"=w161:i32)
              n67 = Equal?(x=w161, y=w160) -> (x = y?=w159:bool)
            }
            n68 = Unbundle By Name(w145) -> ("assets"=w144:T5[])
            n69 = for {
              tunnel: w144 -> [w157] mode=indexing
              tunnel: [w155] -> w139 mode=indexing
              i -> [w153]
              n70 = Unbundle By Name(w157) -> ("slug"=w156:string)
              n71 = Bundle By Name(cluster=cluster{"String":string, "Value":u16} {"String"="", "Value"=0} ("Cluster"), "String"=w156, "Value"=w153) -> (w155:cluster{"String":string, "Value":u16})
            }
            n72 = Bundle By Name(cluster=w151, "InfoStep"=w149) -> (w150:T9)
            n73 = property on="Property Node" class="Ring (strict)"(reference=w138, error in=w141, "StringsAndValues[]"=w139, "Value"=0) -> (error out=w140:errorcluster)  [unwired: 1 out]
          }
          event "Channels": Value Change {
            n74 = event-data() -> ("NewVal"=w162:cluster{"Channel Name":string, "Delete":bool}[])  [unwired: 1 in, 5 out]
            n75 = for {
              tunnel: w162 -> [w173] mode=indexing
              tunnel: [w172] -> w164
              tunnel: [w171] -> w163
              i -> [w171]
              stop <- w172 stop-if-true
              n76 = Unbundle By Name(w173) -> ("Delete"=w172:bool)
            }
            n77 = case shown="True" w164 {
              tunnel: w163 -> [_ w169]
              tunnel: w162 -> [_ w170]
              frame False {
              }
              frame True {
                n78 = Delete From Array(array=w170, index=w169) -> (array with subset deleted=w168:cluster{"Channel Name":string, "Delete":bool}[])  [unwired: 1 in, 1 out]
                n79 = local write "Channels"(w168) -> ()
              }
            }
          }
          event "Inizia Test": Value Change {
            n80 = event-data() -> ()  [unwired: 1 in, 6 out]
          }
          event "Home": Value Change {
            n81 = event-data() -> ()  [unwired: 1 in, 6 out]
          }
          event "Start": Value Change {
            n82 = event-data() -> ()  [unwired: 1 in, 6 out]
            n83 = Unbundle By Name(w183) -> ("queue out"=w182:refnum<queue>)
            n84 = call <vilib>:"Enqueue.vi"("error in (no error)"=w185, "message"="Acquire", "queue in"=w182) -> ("error out"=w184:errorcluster)  [unwired: 6 in, 2 out]
          }
          event "Stop": Value Change {
            n85 = event-data() -> ()  [unwired: 1 in, 6 out]
            n86 = Unbundle By Name(w189) -> ("queue out"=w188:refnum<queue>)
            n87 = call <vilib>:"Enqueue.vi"("error in (no error)"=w191, "message"="Stop", "queue in"=w188) -> ("error out"=w190:errorcluster)  [unwired: 6 in, 2 out]
          }
          event "LogSingle": Value Change {
            n88 = event-data() -> ()  [unwired: 1 in, 6 out]
          }
          event "Begin Acq": Value Change {
            n89 = event-data() -> ()  [unwired: 1 in, 6 out]
          }
          event "Exit": Value Change {
            n90 = event-data() -> ()  [unwired: 1 in, 6 out]
            n91 = Unbundle By Name(w200) -> ("queue out"=w199:refnum<queue>)
            n92 = call <vilib>:"Enqueue.vi"("error in (no error)"=w202, "message"="Exit", "queue in"=w199) -> ("error out"=w201:errorcluster)  [unwired: 6 in, 2 out]
          }
        }
      }
      frame "GetLimsTestsForBench" {
        n93 = Unbundle By Name(w234) -> ("Home.Workstation"=w205:refnum<vi>, "Home"=w233:T8, "Test"=w227:T6, "Test.Select Test"=w216:refnum<vi>)
        n94 = Unbundle By Name(w222) -> ("Workstation"=w204:u16, "Starting Date"=w220:timestamp)
        n95 = Unbundle By Name(w219) -> ("ByteQXAPIBase in"=w231:refnum<class "ByteQXAPIBase.lvclass">)
        n96 = Type Cast(type=refnum<vi>[] [] ("Controls"), x=w233) -> (*(type *) &x=w226:refnum<vi>[])
        n97 = call "GetStringFromRing.vi"("error in (no error)"=w221, "Select Asset"=w204, "Ring in"=w205) -> ("error out"=w207:errorcluster, "String"=w206:string)  [unwired: 7 in]
        n98 = Type Cast(type=w226, x=w227) -> (*(type *) &x=w225:refnum<vi>[])
        n99 = call "ControlVisibility.vi"("error in (no error)"=w207, "Visible"=FALSE, "Controls"=w226) -> ("error out"=w228:errorcluster)  [unwired: 8 in]
        n100 = call "ControlVisibility.vi"("error in (no error)"=w228, "Visible"=TRUE, "Controls"=w225) -> ("error out"=w223:errorcluster)  [unwired: 8 in]
        n101 = call-dynamic "GetLimsTestsForBench.vi"("error in (no error)"=w223, "creation date"=w220, "workbench"=w206, "ByteQXAPIBase in"=w231) -> ("error out"=w212:errorcluster, "list of tests"=w210:T7[], "ByteQXAPIBase out"=w218:refnum<class "ByteQXAPIBase.lvclass">)  [unwired: 5 in]
        n102 = for {
          tunnel: [w241] -> w215 mode=indexing
          tunnel: w210 -> [w240] mode=indexing
          n103 = Unbundle By Name(w240) -> ("titolo"=w237:string, "id"=w242:i32, "slug"=w239:string)
          n104 = Concatenate Strings(w239, " - " ("string"), w237) -> (w236:string)
          n105 = Bundle By Name(cluster=cluster{"String":string, "Value":u16} {"String"="", "Value"=0} ("Cluster"), "String"=w236, "Value"=w242) -> (w241:cluster{"String":string, "Value":u16})
        }
        n106 = Index Array(array=w215) -> (element=w214:cluster{"String":string, "Value":u16})  [unwired: 1 in]
        n107 = Unbundle By Name(w214) -> ("Value"=w208:u16)
        n108 = call "InfoTest.vi"("error in"=w212, "Seleziona Test"=w208, "TestForBenchArray"=w210) -> ("error out"=w211:errorcluster, "Info Test"=w209:string)  [unwired: 7 in]
        n109 = Bundle By Name(cluster=w219, "ByteQXAPIBase in"=w218, "Array dei Test"=w210, "InfoTest"=w209) -> (w217:T9)
        n110 = property on="Property Node" class="Ring (strict)"(reference=w216, error in=w211, "StringsAndValues[]"=w215, "Value"=w208) -> (error out=w213:errorcluster)  [unwired: 1 out]
      }
      frame "GetLimsTestSteps" {
        n111 = Unbundle By Name(w264) -> ("ByteQXAPIBase in"=w261:refnum<class "ByteQXAPIBase.lvclass">)
        n112 = Unbundle By Name(w265) -> ("Select Test"=w260:i32)
        n113 = Unbundle By Name(w257) -> ("Test.Select Step"=w256:refnum<vi>, "Test.Select Asset"=w247:refnum<vi>)
        n114 = call-dynamic "GetLimsTestSteps.vi"("error in (no error)"=w262, "test-id"=w260, "ByteQXAPIBase in"=w261) -> ("error out"=w252:errorcluster, "list of steps"=w255:T4[], "ByteQXAPIBase out"=w259:refnum<class "ByteQXAPIBase.lvclass">)  [unwired: 6 in]
        n115 = for {
          tunnel: [w273] -> w250 mode=indexing
          tunnel: w255 -> [w271] mode=indexing
          tunnel: [w267] -> w246 mode=indexing
          n116 = Unbundle By Name(w271) -> ("descrizione"=w270:string, "id"=w269:i32, "assets"=w268:T5[])
          n117 = for {
            tunnel: w268 -> [w278] mode=indexing
            tunnel: [w276] -> w267 mode=indexing
            i -> [w274]
            n118 = Unbundle By Name(w278) -> ("slug"=w277:string)
            n119 = Bundle By Name(cluster=cluster{"String":string, "Value":u16} {"String"="", "Value"=0} ("Cluster"), "String"=w277, "Value"=w274) -> (w276:cluster{"String":string, "Value":u16})
          }
          n120 = Bundle By Name(cluster=cluster{"String":string, "Value":u16} {"String"="", "Value"=0} ("Cluster"), "String"=w270, "Value"=w269) -> (w273:cluster{"String":string, "Value":u16})
        }
        n121 = Index Array(array=w250) -> (element=w258:cluster{"String":string, "Value":u16})  [unwired: 1 in]
        n122 = Unbundle By Name(w258) -> ("Value"=w251:u16)
        n123 = property on="Property Node" class="Ring (strict)"(reference=w256, error in=w252, "StringsAndValues[]"=w250, "Value"=w251) -> (error out=w249:errorcluster)  [unwired: 1 out]
        n124 = Index Array(array=w246, index (row)=0 ("disabled index (col)")) -> (element=w245:cluster{"String":string, "Value":u16}[])  [unwired: 1 in]
        n125 = property on="Property Node" class="Ring (strict)"(reference=w247, error in=w249, "StringsAndValues[]"=w245, "Value"=0) -> (error out=w248:errorcluster)  [unwired: 1 out]
        n126 = call "infoStepMini.vi"("error in (no error)"=w248, "StepId"=w251, "Array"=w255) -> ("error out"=w254:errorcluster, "Info Test"=w253:string)  [unwired: 7 in]
        n127 = Bundle By Name(cluster=w264, "ByteQXAPIBase in"=w259, "Steps Array"=w255, "InfoStep"=w253) -> (w263:T9)
      }
      frame "GetChannels" {
        n128 = Unbundle By Name(w291) -> ("Test.Select Asset"=w290:refnum<vi>)
        n129 = Unbundle By Name(w289) -> ("Select Asset"=w288:i32)
        n130 = Unbundle By Name(w285) -> ("ByteQXAPIBase in"=w293:refnum<class "ByteQXAPIBase.lvclass">)
        n131 = call "GetStringFromRing.vi"("error in (no error)"=w292, "Select Asset"=w288, "Ring in"=w290) -> ("error out"=w286:errorcluster, "String"=w287:string)  [unwired: 7 in]
        n132 = call "GetChannelList.vi"("error in (no error)"=w286, "asset code"=w287, "ByteGSAPIBase in"=w293) -> ("error out"=w282:errorcluster, "channels"=w280:string[], "ByteGSAPIBase out"=w283:refnum<class "ByteQXAPIBase.lvclass">)  [unwired: 6 in]
        n133 = for {
          tunnel: w280 -> [w295] mode=indexing
          tunnel: [w294] -> w279 mode=indexing
          n134 = Bundle By Name(cluster=cluster{"Channel Name":string, "Home":bool} {"Channel Name"="", "Home"=FALSE} ("Channels"), "Channel Name"=w295) -> (w294:cluster{"Channel Name":string, "Home":bool})
        }
        n135 = local write "Channels"(w279) -> ()
        n136 = Bundle By Name(cluster=w285, "ByteQXAPIBase in"=w283) -> (w284:T9)
      }
      frame "UpdateChannels" {
        n137 = Unbundle By Name(w311) -> ("Channels"=w309:cluster{"Channel Name":string, "Delete":bool}[], "Select Asset"=w304:i32)
        n138 = Unbundle By Name(w301) -> ("ByteQXAPIBase in"=w310:refnum<class "ByteQXAPIBase.lvclass">)
        n139 = for {
          tunnel: w309 -> [w313] mode=indexing
          tunnel: [w312] -> w308 mode=indexing
          n140 = Unbundle By Name(w313) -> ("Channel Name"=w312:string)
        }
        n141 = Unbundle By Name(w306) -> ("Test.Select Asset"=w305:refnum<vi>)
        n142 = call "GetStringFromRing.vi"("error in (no error)"=w307, "Select Asset"=w304, "Ring in"=w305) -> ("error out"=w303:errorcluster, "String"=w302:string)  [unwired: 7 in]
        n143 = call "UpdateChannelsList.vi"("error in (no error)"=w303, "channels"=w308, "asset code"=w302, "ByteQXAPIBase in"=w310) -> ("error out"=w298:errorcluster, "ByteQXAPIBase out"=w299:refnum<class "ByteQXAPIBase.lvclass">)  [unwired: 6 in]
        n144 = Bundle By Name(cluster=w301, "ByteQXAPIBase in"=w299) -> (w300:T9)
      }
      frame "StartTest" {
        n145 = Unbundle By Name(w351) -> ("Home.Workstation"=w347:refnum<vi>, "Test.Select Test"=w343:refnum<vi>, "Test.Select Step"=w341:refnum<vi>, "Test.Select Asset"=w339:refnum<vi>, "Test"=w359:T6, "Running"=w355:T3)  [unwired: 1 out]
        n146 = Unbundle By Name(w349) -> ("Channels"=w329:cluster{"Channel Name":string, "Delete":bool}[], "Select Asset"=w338:i32, "Select Step"=w320:i32, "Select Test"=w344:i32, "Workstation"=w346:u16)
        n147 = call "GetStringFromRing.vi"("Index"=TRUE, "error in (no error)"=w348, "Select Asset"=w346, "Ring in"=w347) -> ("error out"=w345:errorcluster, "String"=w334:string)  [unwired: 6 in]
        n148 = call "GetStringFromRing.vi"("error in (no error)"=w345, "Select Asset"=w344, "Ring in"=w343) -> ("error out"=w342:errorcluster, "String"=w333:string)  [unwired: 7 in]
        n149 = call "GetStringFromRing.vi"("error in (no error)"=w342, "Select Asset"=w320, "Ring in"=w341) -> ("error out"=w340:errorcluster, "String"=w332:string)  [unwired: 7 in]
        n150 = Unbundle By Name(w316) -> ("ByteQXAPIBase in"=w324:refnum<class "ByteQXAPIBase.lvclass">, "Steps Array"=w321:T4[])
        n151 = call "GetStringFromRing.vi"("Index"=TRUE, "error in (no error)"=w340, "Select Asset"=w338, "Ring in"=w339) -> ("error out"=w337:errorcluster, "String"=w322:string)  [unwired: 6 in]
        n152 = Type Cast(type=refnum<vi>[] [] ("Controls"), x=w359) -> (*(type *) &x=w354:refnum<vi>[])
        n153 = Format Into String(format string="%s - %s - %s - %s", error in=w337, w334, w333, w332, w322) -> (resulting string=w314:string, error out=w336:errorcluster)  [unwired: 1 in]
        n154 = for {
          tunnel: w321 -> [w364] mode=indexing
          tunnel: w320 -> [w362]
          tunnel: [w361] -> w319
          stop <- w360 stop-if-true
          n155 = Unbundle By Name(w364) -> ("prova.slug"=w361:string, "id"=w363:i32)
          n156 = Equal?(x=w363, y=w362) -> (x = y?=w360:bool)
        }
        n157 = for {
          tunnel: w329 -> [w366] mode=indexing
          tunnel: [w365] -> w323 mode=indexing
          n158 = Unbundle By Name(w366) -> ("Channel Name"=w365:string)
        }
        n159 = Type Cast(type=w354, x=w355) -> (*(type *) &x=w353:refnum<vi>[])
        n160 = call "ControlVisibility.vi"("error in (no error)"=w336, "Visible"=FALSE, "Controls"=w354) -> ("error out"=w356:errorcluster)  [unwired: 8 in]
        n161 = call "ControlVisibility.vi"("error in (no error)"=w356, "Visible"=TRUE, "Controls"=w353) -> ("error out"=w328:errorcluster)  [unwired: 8 in]
        n162 = Bundle By Name(cluster=w316, "Title"=w314) -> (w315:T9)
        n163 = Bundle(cluster=T13 {"ByteQXAPIBase in"=refnum, "slug"="", "Channels"=[], "Step Id"=0, "AssetCode"=""}, "ByteQXAPIBase in"=w324, "slug"=w319, "Channels"=w323, "Step Id"=w320, "AssetCode"=w322) -> (w318:T13)
        n164 = Unbundle By Name(w315) -> ("queue out"=w327:refnum<queue>)
        n165 = call <vilib>:"Enqueue.vi"("error in (no error)"=w328, "data"=w318, "message"="Setup", "queue in"=w327) -> ("error out"=w325:errorcluster)  [unwired: 5 in, 2 out]
      }
      frame "GetAsset" {
        n166 = Unbundle By Name(w387) -> ("Asset Code"=w367:string)
        "Single Asset" <- w367
        n167 = Unbundle By Name(w383) -> ("ByteQXAPIBase in"=w384:refnum<class "ByteQXAPIBase.lvclass">)
        n168 = Unbundle By Name(w376) -> ("Home"=w374:T8, "Single"=w373:T2)
        n169 = Type Cast(type=refnum<vi>[] [] ("Controls"), x=w374) -> (*(type *) &x=w372:refnum<vi>[])
        n170 = call "ControlVisibility.vi"("error in (no error)"=w378, "Visible"=FALSE, "Controls"=w372) -> ("error out"=w371:errorcluster)  [unwired: 8 in]
        n171 = Type Cast(type=w372, x=w373) -> (*(type *) &x=w370:refnum<vi>[])
        n172 = call "ControlVisibility.vi"("error in (no error)"=w371, "Visible"=TRUE, "Controls"=w370) -> ("error out"=w368:errorcluster)  [unwired: 8 in]
        n173 = call "GetChannelList.vi"("error in (no error)"=w368, "asset code"=w367, "ByteGSAPIBase in"=w384) -> ("error out"=w385:errorcluster, "channels"=w386:string[], "ByteGSAPIBase out"=w381:refnum<class "ByteQXAPIBase.lvclass">)  [unwired: 6 in]
        n174 = for {
          tunnel: w386 -> [w389] mode=indexing
          tunnel: [w388] -> w380 mode=indexing
          n175 = Bundle By Name(cluster=cluster{"Channel Name":string, "Home":bool} {"Channel Name"="", "Home"=FALSE} ("Channels"), "Channel Name"=w389) -> (w388:cluster{"Channel Name":string, "Home":bool})
        }
        n176 = local write "Channels"(w380) -> ()
        n177 = Bundle By Name(cluster=w383, "ByteQXAPIBase in"=w381) -> (w382:T9)
      }
      frame "StartSingle" {
        n178 = Unbundle By Name(w404) -> ("Asset Code"=w394:string, "Channels"=w392:cluster{"Channel Name":string, "Delete":bool}[])
        n179 = Unbundle By Name(w410) -> ("Single"=w408:T2, "Running"=w407:T3)
        n180 = Type Cast(type=refnum<vi>[] [] ("Controls"), x=w408) -> (*(type *) &x=w406:refnum<vi>[])
        n181 = Type Cast(type=w406, x=w407) -> (*(type *) &x=w405:refnum<vi>[])
        n182 = for {
          tunnel: w392 -> [w416] mode=indexing
          tunnel: [w415] -> w391 mode=indexing
          n183 = Unbundle By Name(w416) -> ("Channel Name"=w415:string)
        }
        n184 = call "ControlVisibility.vi"("error in (no error)"=w411, "Visible"=FALSE, "Controls"=w406) -> ("error out"=w413:errorcluster)  [unwired: 8 in]
        n185 = call "ControlVisibility.vi"("error in (no error)"=w413, "Visible"=TRUE, "Controls"=w405) -> ("error out"=w400:errorcluster)  [unwired: 8 in]
        n186 = Unbundle By Name(w399) -> ("queue out"=w398:refnum<queue>, "ByteQXAPIBase in"=w395:refnum<class "ByteQXAPIBase.lvclass">)
        n187 = Bundle By Name(cluster=T13 {"ByteQXAPIBase in"=refnum, "slug"="", "Channels"=[], "Step Id"=0, "AssetCode"=""}, "ByteQXAPIBase in"=w395, "AssetCode"=w394, "Channels"=w391) -> (w393:T13)
        n188 = Bundle By Name(cluster=w399, "Title"=w394) -> (w403:T9)
        n189 = call <vilib>:"Enqueue.vi"("error in (no error)"=w400, "data"=w393, "message"="Setup", "queue in"=w398) -> ("error out"=w397:errorcluster)  [unwired: 5 in, 2 out]
      }
    }
    n190 = Unbundle By Name(w59) -> ("InfoTest"=→"InfoTest":string, "InfoStep"=→"InfoStep":string, "Title"=→"Title":string)
  }
  n191 = while {
    shift-right: [w421] -> _
    shift-left: w22 -> [w423]
    tunnel: w21 -> [w429]
    tunnel: errorcluster {"status"=FALSE, "code"=0, "source"=""} ("error in (no error)") -> [w428]
    tunnel: [w422] -> w9
    stop <- w424 stop-if-true
    n192 = call <vilib>:"Dequeue.vi"("error in (no error)"=w428, "queue in"=w429) -> ("error out"=w427:errorcluster, "data"=w426:variant, "message"=w425:string, "queue out"=w419:refnum<queue>)  [unwired: 5 in, 1 out]
    n193 = case shown="\"Acquire\"" w425 {
      tunnel: w427 -> [w431 w432 w451 w475 w489 w492]
      tunnel: w426 -> [_ _ w450 _ _ _]
      tunnel: [_ _ _ _ _ TRUE] -> w424
      tunnel: w423 -> [w430 w435 w449 w480 w490 w491]
      tunnel: [w430 w433 w439 w479 w490 w491] -> w421
      tunnel: [w431 w432 w440 w478 w487 w492] -> w422
      tunnel: w419 -> [_ _ _ w477 w488 _]
      frame Default {
      }
      frame "Init" {
        n194 = Bundle By Name(cluster=w435, "Values"=cluster{"Channel Name":string, "Value":dbl}[] []) -> (w433:T11)
      }
      frame "Setup" {
        n195 = Variant To Data(error in=w451, type=T13 {"ByteQXAPIBase in"=refnum, "slug"="", "Channels"=[], "Step Id"=0, "AssetCode"=""} ("cluster"), Variant=w450) -> (data=w446:T13, error out=w441:errorcluster)
        n196 = Unbundle By Name(w446) -> ("ByteQXAPIBase in"=w445:refnum<class "ByteQXAPIBase.lvclass">, "slug"=w444:string, "Channels"=w437:string[], "Step Id"=w443:i32, "AssetCode"=w442:string)
        n197 = for {
          tunnel: w437 -> [w461] mode=indexing
          tunnel: [w460] -> w448 mode=indexing
          n198 = Bundle By Name(cluster=cluster{"Channel Name":string, "Value":dbl} {"Channel Name"="", "Value"=0.0} ("Cluster 2"), "Channel Name"=w461) -> (w460:cluster{"Channel Name":string, "Value":dbl})
        }
        n199 = Bundle By Name(cluster=w449, "ByteQXAPIBase in"=w445, "slug"=w444, "Values"=w448, "Step Id"=w443, "AssetCode"=w442) -> (w439:T11)
        n200 = Unbundle By Name(w439) -> ("Waveform Chart"=w438:refnum<vi>)
        n201 = for {
          N: 50 -> [_]
          tunnel: w441 -> [w459]
          tunnel: [w458] -> w440
          tunnel: w438 -> [w457]
          tunnel: w437 -> [w455]
          i -> [w456]
          n202 = Index Array(array=w455, index=w456) -> (element=w454:string)
          n203 = Empty String/Path?(string/path=w454) -> (empty?=w453:bool)
          n204 = Not(x=w453) -> (.not. x?=w452:bool)
          n205 = property class="WFChart (strict)"(reference=w457, error in=w459, "Active Plot"=w456, "Plot.Plot Name"=w454, "Plot.Visible?"=w452) -> (error out=w458:errorcluster)  [unwired: 1 out]
        }
      }
      frame "Acquire" {
        n206 = Unbundle By Name(w480) -> ("Values"=w481:cluster{"Channel Name":string, "Value":dbl}[], "Step Id"=w471:i32, "ByteQXAPIBase in"=w473:refnum<class "ByteQXAPIBase.lvclass">, "AssetCode"=w470:string, "slug"=w469:string)
        n207 = for {
          tunnel: w481 -> [w485] mode=indexing
          tunnel: [w484] -> w466 mode=indexing
          tunnel: [w483] -> w463 mode=indexing
          n208 = call-poly <vilib>:"Random Number (Range).vi"("upper bound (100)"=u64 500) -> ("number"=w483:u64)  [unwired: 10 in]
          n209 = Bundle By Name(cluster=w485, "Value"=w483) -> (w484:cluster{"Channel Name":string, "Value":dbl})
        }
        n210 = Get Date/Time In Seconds() -> (seconds since 1Jan1904=w467:timestamp)
        n211 = Bundle By Name(cluster=T15 {"timestamp"=timestamp(0 s since 1904-01-01), "channels"=[]} ("acquisitions"), "timestamp"=w467, "channels"=w466) -> (w465:T15)
        n212 = Build Array(w465) -> (w464:T15[])
        n213 = Wait (ms)(milliseconds to wait=u32 500) -> ()  [unwired: 1 out]
        n214 = call-dynamic "UploadAcquisitions.vi"("test slug"=w469, "step id"=w471, "error in (no error)"=w475, "acquisitions"=w464, "asset code"=w470, "ByteQXAPIBase in"=w473) -> ("error out"=w474:errorcluster, "ByteQXAPIBase out"=w472:refnum<class "ByteQXAPIBase.lvclass">)  [unwired: 4 in]
        n215 = Bundle By Name(cluster=w480, "Graph"=w463, "Values"=w466, "ByteQXAPIBase in"=w472) -> (w479:T11)
        n216 = call <vilib>:"Enqueue.vi"("error in (no error)"=w474, "message"="Acquire", "queue in"=w477) -> ("error out"=w478:errorcluster)  [unwired: 6 in, 2 out]
      }
      frame "Stop" {
        n217 = call <vilib>:"Flush.vi"("error in"=w489, "queue in"=w488) -> ("error out"=w487:errorcluster)  [unwired: 8 in, 1 out]
      }
      frame "Exit" {
      }
    }
    n218 = Unbundle By Name(w421) -> ("Values"=→"Values":cluster{"Channel Name":string, "Value":dbl}[], "Graph"=w418:u64[])
    n219 = Array To Cluster(array=w418) -> (cluster=→"Waveform Chart":T1)
  }
  n220 = Merge Errors(w10, w9) -> ()  [unwired: 1 out]
